vi "Create Header Contents.vi"(8 "error in (no error)":errorcluster, 11 "Setup File in":refnum<class "Setup File.lvclass">) -> (0 "error out":errorcluster, 3 "Setup File out":refnum<class "Setup File.lvclass">)   [LabVIEW 2012, in "Setup File.lvclass"]
uses:
  Setup File.lvclass
  Setup File.lvclass/Setup File.ctl
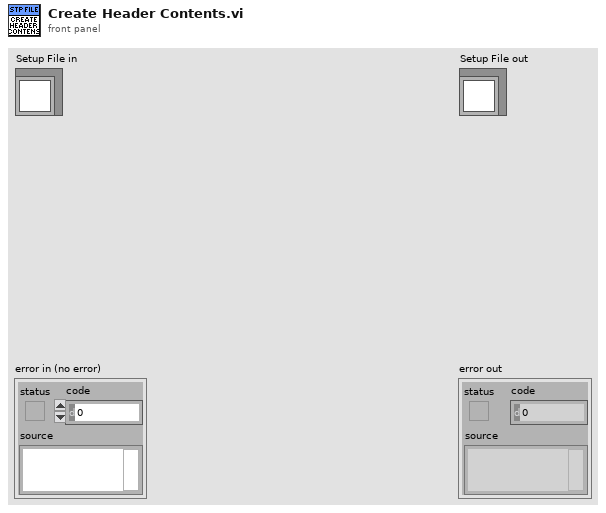
[diagram p1: front panel]
types:
  T1 = enum16{"open", "replace", "create", "open or create", "replace or create", "replace or create with confirmation"}
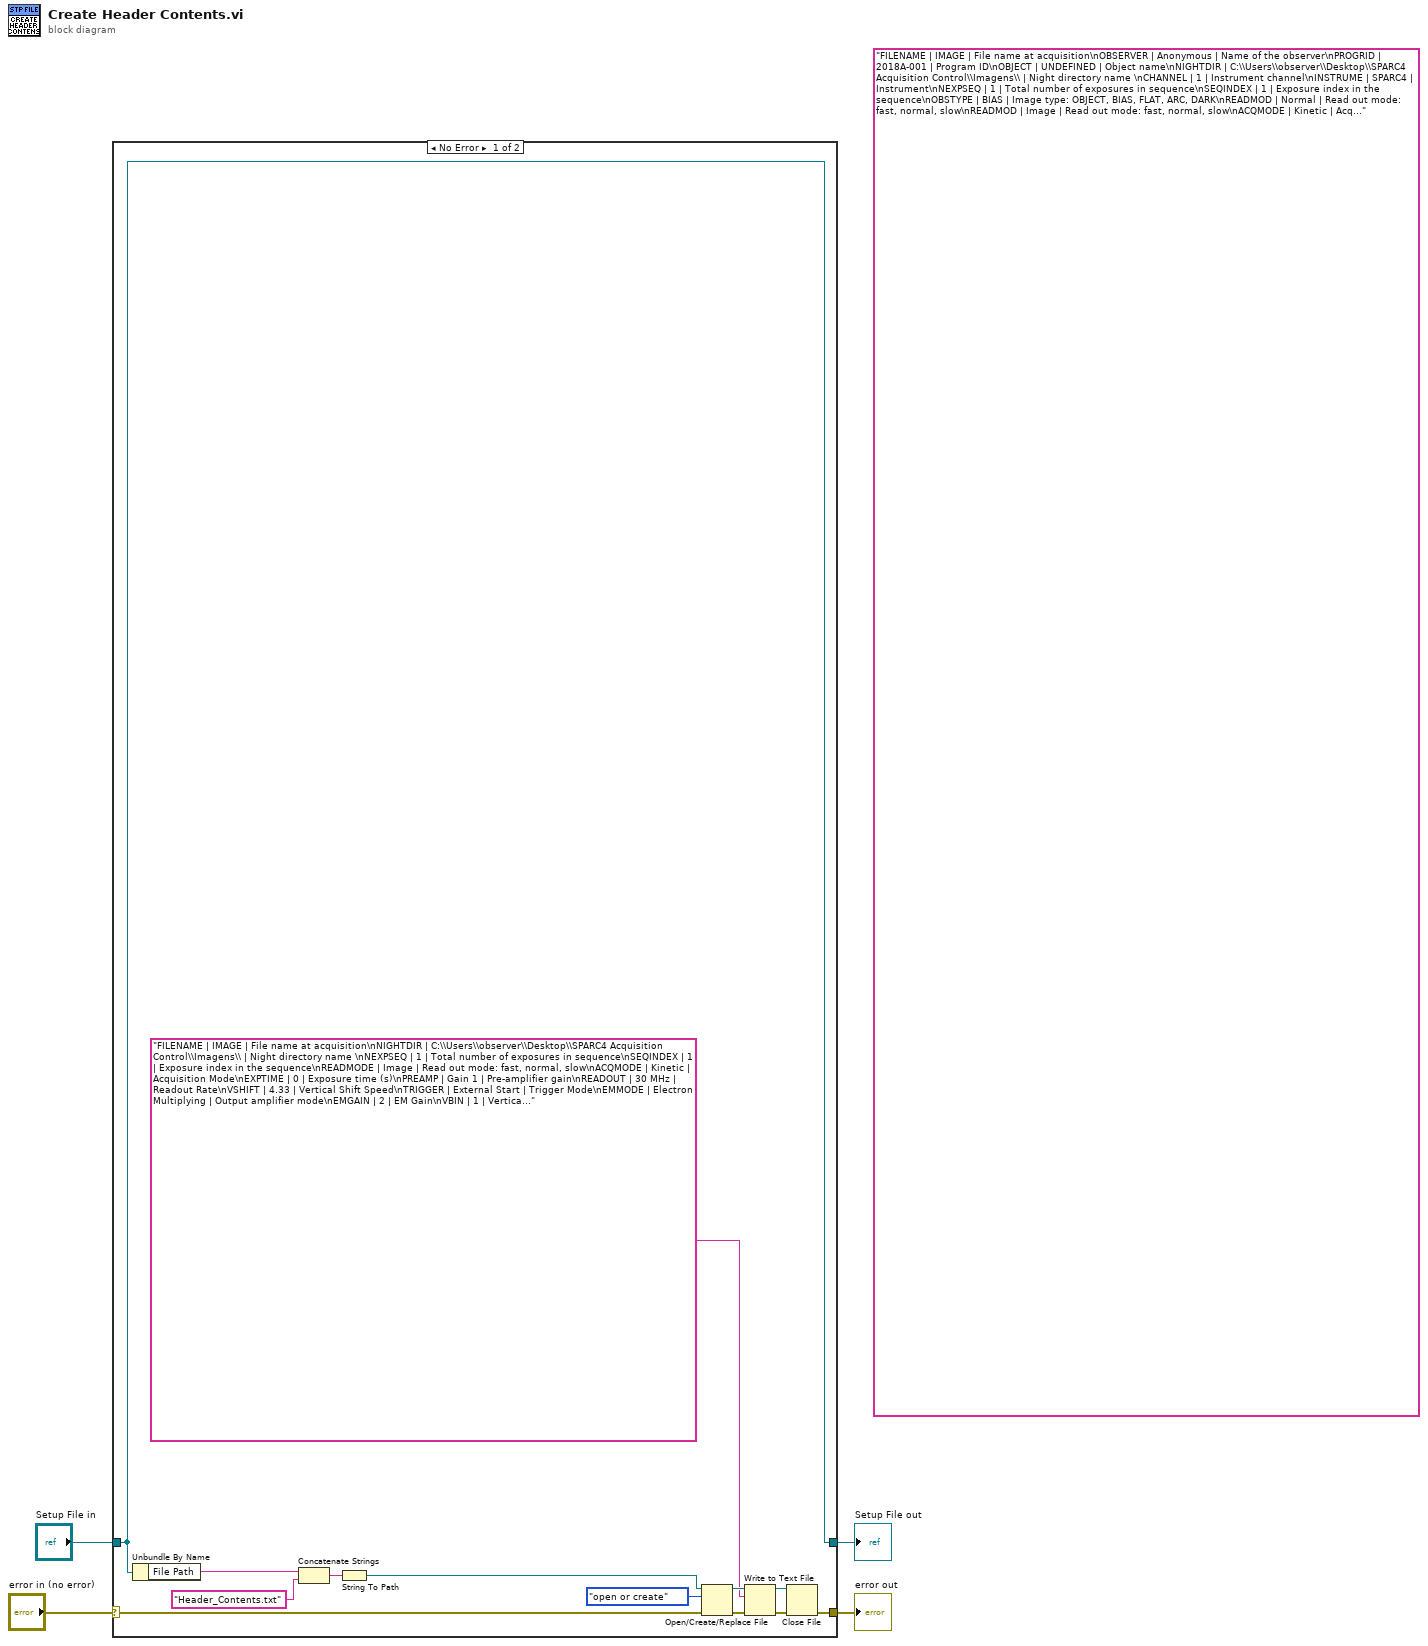
[diagram p0: block diagram]
diagram:
  (unwired) "FILENAME | IMAGE | File name at acquisition\nOBSERVER | Anonymous | Name of the observer\nPROGRID | 2018A-001 | Program ID\nOBJECT | UNDEFINED | Object name\nNIGHTDIR | C:\\Users\\observer\\Desktop\\SPARC4 Acquisition Control\\Imagens\\ | Night directory name \nCHANNEL | 1 | Instrument channel\nINSTRUME | SPARC4 | Instrument\nNEXPSEQ | 1 | Total number of exposures in sequence\nSEQINDEX | 1 | Exposure index in the sequence\nOBSTYPE | BIAS | Image type: OBJECT, BIAS, FLAT, ARC, DARK\nREADMOD | Normal | Read out mode: fast, normal, slow\nREADMOD | Image | Read out mode: fast, normal, slow\nACQMODE | Kinetic | Acquisition Mode\nEXPTIME | 0 | Exposure time (s)\nPREAMP | Gain 1 | Pre-amplifier gain\nREADOUT | 30 MHz | Readout Rate\nVSHIFT | 4.33 | Vertical Shift Speed\nTRIGGER | Internal | Trigger Mode\nEMMODE | Electron Multiplying | Output amplifier mode\nEMGAIN | 2 | EM Gain\nVBIN | 1 | Vertical binning\nHBIN | 1 | Horizontal binning\nINITLIN | 1 | Initial Line\nINITCOL | 1 | Initial Column\nFINALLIN | 1024 | Final Line\nFINALCOL | 1024 | Final Column\nKSERLEN | 1 | Kinetic Series Length\nSHUTTER | CLOSED | Shutter Mode (OPEN, CLOSED, or AUTO) \nSHTTTL | TTL LOW | Shutter TTL\nOPENSHT | 50 | Time to open the shutter (ms) \nCLOSESHT | 50 | Time to close the shutter (ms)\nDATE | 2019-03-14T17:16:54.78 | Date of the acquired image (YY/MM/DD:HH:MM:SS.sss)\nGAIN | 3.38 | Gain (e-/ADU)\nGAINERR | 0.05 |  Gain error (e-/ADU)\nRDNOISE | 6.55 | Read noise (e-)\nRNOISERR | 0.02 | Read noise error (e-)\nSKYFIBER | \"OFF\" | Sky fiber: ON or OFF\nCALFIBER | \"OFF\" | Calibration Fiber: ON or OFF\nUTDATE | '2017-10-01T20 | UT date at start of exposure\nLOCTIME | '2017-10-01T17 | LT date at start of exposure\nMJD | 58027.500000 | Modified Julian Date at start of exposure\nOBSLON | -45.57972 | Observatory East Longitude\nOBSLAT | -22.53444 | Observatory Latitude\nOBSALT | 1864.0 | Observatory elevation above sea level (m)\nTELRA | “00:00:00.000” | TCS right ascension: HH:MM:SS.SSS\nTELDEC | “+00:00:00.000” | TCS declination: +-DD:MM:SS.SSS\nRA | “00:00:00.000” | Requested right Ascension: HH:MM:SS.SSS\nDEC | “+00:00:00.000” | Requested Declination: +- DD:MM:SS.SSS\nRA_DEG | 128.84946 | Requested Right Ascension (deg)\nDEC_DEG | +19.648717 | Requested Declination (deg)\nEPOCH | 2000.00 | Epoch for Target coordinates\nHA | “+01:13:05.98” | Hour Angle (Sexagesimal)\nHAD | 1.2183292 | Hour Angle (deg)\nAIRMASS | 1.085 | Mean airmass for the observation\nAMSTART | 1.060 | Airmass at start of exposure\nAMEND | 1.114 | Airmass at end of exposure\nXOFFSET | 0.000000 | Telescope RA offset in arcsec\nYOFFSET | 0.000000 | Telescope DEC offset in arcsec\nPA | 14.6415392418 | Current Rotator Position Angle (degree)\nCAMFOC | -3.53 | Camera focus position (mm)\nTELFOC | -3.53 | Telescope focus position (mm)\nTCSUT | ‘23:17:24.8’ | TCS Universal Time\nTCSST | ‘23:12:32.5’ | TCS Sideral Time\nMOONDIST | 60.0 | Moon angular distance to object (deg)\nMOONALT | 15.0 | Moon elevation above horizon (deg)\nMOONPHAS | 30.0 | Moon phase (deg)\nADC | OFF | Atmospheric Dispersion Corrector: ON or OFF\nADCSPEED | 0 | ADC motor speed (rpm)\nCALMIRR | \"OUT\" | Calibration mirror position: IN or OUT\nGUIDING | OFF | Guider status: ON or OFF\nGUIDTEXP | 0 | Guider exposure time (s)\nGUIDFREQ | 0 | Guiding frequency (Hz)\nGUIDOBJX | 102.5 | Guiding object x position (pixel)\nGUIDOBJY | 300.3 | Guiding object y position (pixel)\nAVGYCORR | 2.3 | Average correction in RA (arcsec)\nAVGXCORR | 1.3 | Average correction in DEC (arcsec)\nGFOCUS | 3.0 | Guider focus position (mm)\nTHARLAMP | “OFF” | Thorium-Argon lamp state: ON or OFF\nHALLAMP | “OFF” | Halogen lamp state: ON or OFF\nAGITATOR | “OFF” | Fiber agitator: ON or OFF\nTHARMIRR | “SPECTROGRAPH” | Th-Ar mirror position: SPECTROGRAPH or TELESCOPE\nDSTATUS | ‘OPEN’ | Dome Status: OPEN or CLOSED\nDTEMP | 10.0 | Dome temperature (deg C)\nDHUM | 82.0 | Dome humidity (per cent)\nDLAMP | “OFF” | Dome lamp: ON or OFF\nDFLAT | “OFF” | Dome flat lamp: ON or OFF\nTEMPEXT | 10.0 | External temperature (deg C)\nPRESSURE | 742.00 | Pressure (mbar)\nHUMIDITY | 92.00 | Humidity (per cent)\nWINDDIR | 15.0| Wind direction: North-eastward (deg)\nWSPEED | 30.2 | Wind Speed (km/h)"
  n1 = case shown="No Error" "error in (no error)" {
    selector: "error in (no error)" -> [w9 w19]
    tunnel: [w8 w19] -> w3
    tunnel: [w7 w18] -> w1
    tunnel: "Setup File in" -> [w7 w18]
    frame No Error {
      n2 = Unbundle By Name(w7) -> ("File Path"=w5:string)
      n3 = Concatenate Strings(w5, "Header_Contents.txt") -> (w13:string)
      n4 = String To Path(string=w13) -> (path=w12:path)
      n5 = Open/Create/Replace File(file path (use dialog)=w12, error in=w9, operation (0:open)=T1."open or create") -> (refnum out=w15:refnum<file>, error out=w17:errorcluster)  [unwired: 3 in, 1 out]
      n6 = Write to Text File(file (use dialog)=w15, text="FILENAME | IMAGE | File name at acquisition\nNIGHTDIR | C:\\Users\\observer\\Desktop\\SPARC4 Acquisition Control\\Imagens\\ | Night directory name \nNEXPSEQ | 1 | Total number of exposures in sequence\nSEQINDEX | 1 | Exposure index in the sequence\nREADMODE | Image | Read out mode: fast, normal, slow\nACQMODE | Kinetic | Acquisition Mode\nEXPTIME | 0 | Exposure time (s)\nPREAMP | Gain 1 | Pre-amplifier gain\nREADOUT | 30 MHz | Readout Rate\nVSHIFT | 4.33 | Vertical Shift Speed\nTRIGGER | External Start | Trigger Mode\nEMMODE | Electron Multiplying | Output amplifier mode\nEMGAIN | 2 | EM Gain\nVBIN | 1 | Vertical binning\nHBIN | 1 | Horizontal binning\nINITLIN | 1 | Initial Line\nINITCOL | 1 | Initial Column\nFINALLIN | 1024 | Final Line\nFINALCOL | 1024 | Final Column\nKSERLEN | 1 | Kinetic Series Length\nSHUTTER | CLOSED | Shutter Mode (OPEN, CLOSED, or AUTO) \nSHTTTL | TTL LOW | Shutter TTL\nOPENSHT | 50 | Time to open the shutter (ms) \nCLOSESHT | 50 | Time to close the shutter (ms)\nDATE | 2019-03-14T17:16:54.78 | Date of the acquired image (YY/MM/DD:HH:MM:SS.sss)", error in=w17) -> (refnum out=w14:refnum<file>, error out=w16:errorcluster)  [unwired: 1 in, 1 out]
      n7 = Close File(refnum=w14, error in=w16) -> (error out=w8:errorcluster)  [unwired: 1 out]
    }
    frame Error {
    }
  }
  "error out" <- w3
  "Setup File out" <- w1
